vi "nData.vi"(7 "LabVIEW Web Service Request":refnum<class "Web Request.lvclass">) -> ()   [LabVIEW 2014]
uses:
  <vilib>/wsapi/Web Request.lvclass
  Data/Nicholas Data.lvclass
panel:
  # "Use the Web Service Request input terminal to call the VIs on the Web Services palette. Do not remove it from the connector pane unless you don't need access to the palette."
  # "Each additional control wired to the connector pane will be available as an input in the URL. To include an indicator in terminal-mode output (the default setting), it must also be wired to the connector pane."
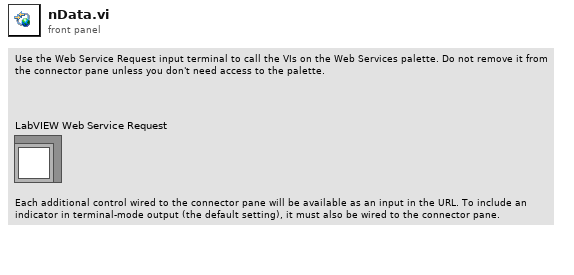
[diagram p1: front panel]
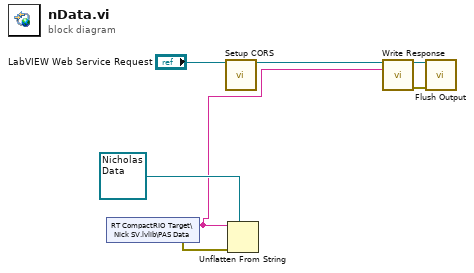
[diagram p0: block diagram]
diagram:
  n1 = shared-variable "RT CompactRIO Target\\Nick SV.lvlib\\PAS Data"() -> (w1:string, error out=w6:errorcluster)  [unwired: 1 in]
  n2 = call "Setup CORS.vi"("Web Request in"="LabVIEW Web Service Request") -> ("Web Request out"=w2:refnum<class "Web Request.lvclass">)  [unwired: 17 in, 1 out]
  n3 = Unflatten From String(type=refnum<class "Nicholas Data.lvclass"> refnum ("nData"), binary string=w1, error in (no error)=w6) -> ()  [unwired: 2 in, 3 out]
  n4 = call <vilib>:"Write Response.vi"("LabVIEW Web Service Request"=w2, "response string"=w1) -> ("LabVIEW Web Service Request out"=w4:refnum<class "Web Request.lvclass">, "error out"=w3:errorcluster)  [unwired: 12 in]
  n5 = call <vilib>:"Flush Output.vi"("LabVIEW Web Service Request"=w4, "error in (no error)"=w3) -> ()  [unwired: 12 in, 2 out]
